vi "Data File Path.vi"() -> (3 "data file path":path)   [LabVIEW 2019, in "Pet Feeder.lvlib"]
uses:
  Pet Feeder.lvlib
  Pet Feeder.vi
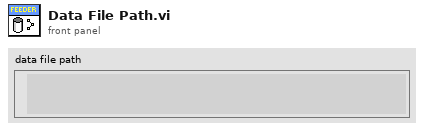
[diagram p1: front panel]
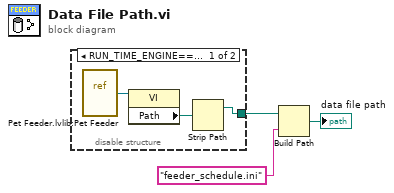
[diagram p0: block diagram]
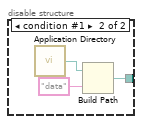
[diagram p2: hidden frame]
diagram:
  n1 = disable-structure shown="RUN_TIME_ENGINE==False" {
    disable-tunnel: [w4 w7] -> w3
    frame condition #0 (active) {
      n2 = vi-ref "Pet Feeder.lvlib:Pet Feeder.vi"() -> (w6:refnum<vi>)
      n3 = property class="VI"(reference=w6) -> ("Path"=w5:path)  [unwired: 1 in, 2 out]
      n4 = Strip Path(path=w5) -> (stripped path=w4:path)  [unwired: 1 out]
    }
    frame condition #1 {
      n5 = call <vilib>:"Application Directory.vi"() -> ("Application Directory"=w9:path)
      n6 = Build Path(base path=w9, name or relative path="data") -> (appended path=w7:path)
    }
  }
  n7 = Build Path(base path=w3, name or relative path="feeder_schedule.ini") -> (appended path=→"data file path":path)
